vi "Teste_freescale.vi"() -> ()   [LabVIEW 2019]
uses:
  <vilib>/Instr/_visa.llb/VISA Configure Serial Port (Instr).vi
panel:
  in  "Escrever para a \nplaca em\n decimal":string
  out "hexadecimal para a placa":string
  out "leitura da placa":string
  in  "VISA resource name":refnum<visa-resource-name>
  in  "stop":bool
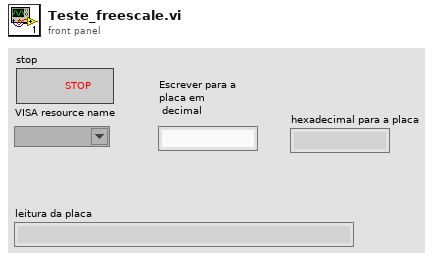
[diagram p1: front panel]
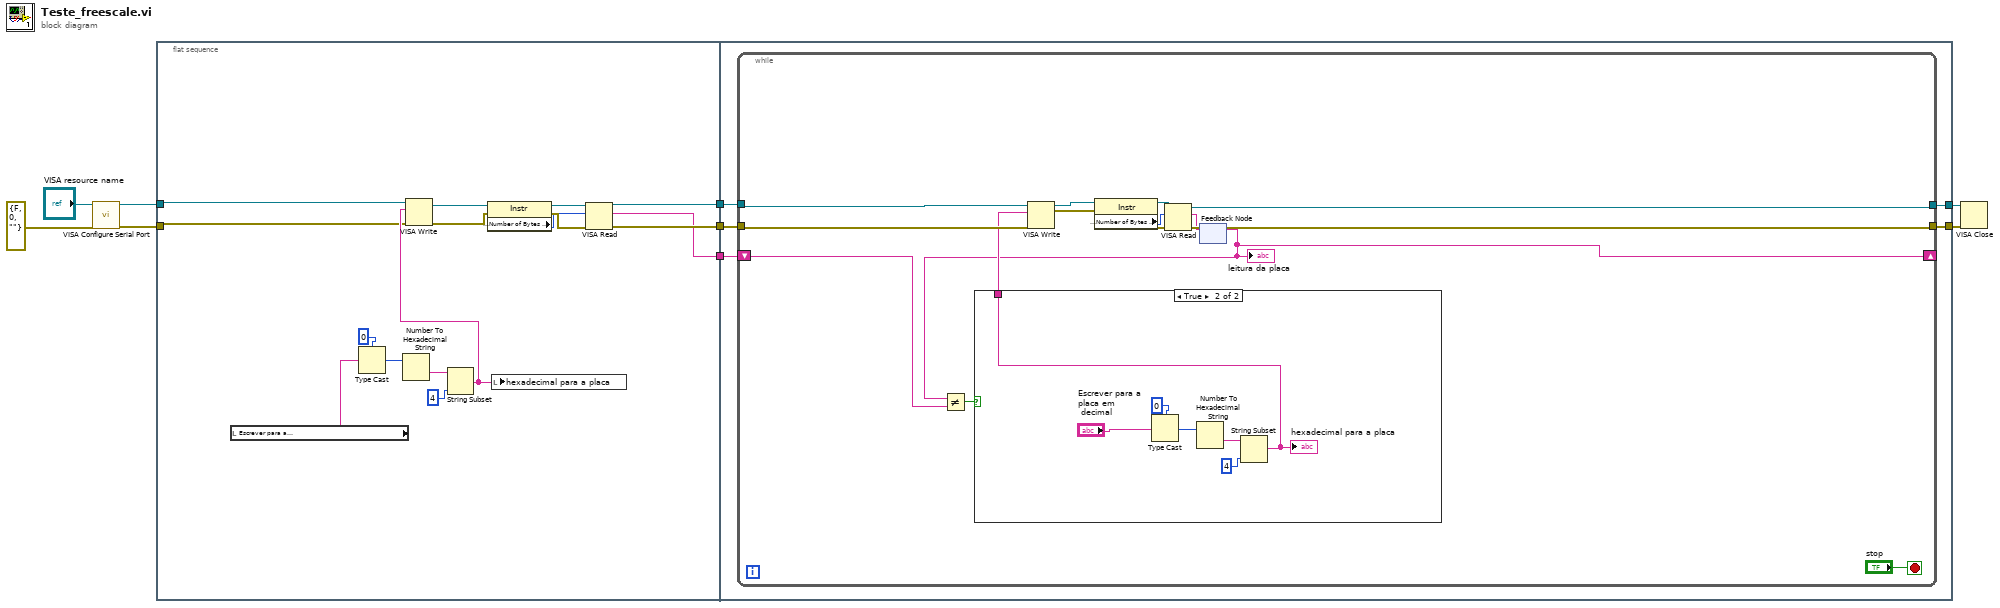
[diagram p0: block diagram]
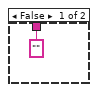
[diagram p2: hidden frame]
diagram:
  n1 = call-poly "VISA Configure Serial Port"("VISA resource name"="VISA resource name", "error in (no error)"=errorcluster {"status"=FALSE, "code"=0, "source"=""}) -> ("VISA resource name out"=w8:refnum<visa-resource-name>, "error out"=w7:errorcluster)  [unwired: 12 in]
  n2 = flat-sequence {
    tunnel: w7 -> [w19]
    tunnel: w8 -> [w18]
    tunnel: [w11] -> w3
    tunnel: [w12] -> w2
    tunnel: [w10] -> w1
    tunnel: [w28] -> w5
    tunnel: [w27] -> w4
    tunnel: w3 -> [w29]
    tunnel: w2 -> [w30]
    tunnel: w1 -> [w26]
    frame #0 {
      n3 = local read "Escrever para a \nplaca em\n decimal"() -> (w21:string)
      n4 = Type Cast(type=0, x=w21) -> (*(type *) &x=w23:i32)
      n5 = Number To Hexadecimal String(2:w23) -> (0:w24:string)  [unwired: 1 in]
      n6 = String Subset(string=w24, length (rest)=4 ("length (rest)")) -> (substring=w20:string)  [unwired: 1 in]
      n7 = VISA Write(VISA resource name=w18, write buffer=w20, error in (no error)=w19) -> (VISA resource name out=w16:refnum<visa-resource-name>, error out=w15:errorcluster)  [unwired: 1 out]
      n8 = property class="Instr"(reference=w16, error in=w15) -> (reference out=w17:refnum<visa-resource-name>, error out=w14:errorcluster, "Serial Settings:Number of Bytes at Serial Port"=w13:u32)
      n9 = local write "hexadecimal para a placa"(w20) -> ()
      n10 = VISA Read(VISA resource name=w17, byte count=w13, error in (no error)=w14) -> (VISA resource name out=w12:refnum<visa-resource-name>, read buffer=w10:string, error out=w11:errorcluster)  [unwired: 1 out]
    }
    frame #1 {
      n11 = while {
        tunnel: w30 -> [w44]
        tunnel: w29 -> [w43]
        tunnel: [w42] -> w28
        tunnel: [w41] -> w27
        shift-right: [w31] -> _
        shift-left: w26 -> [w33]
        stop <- "stop" stop-if-true
        n12 = feedback #1() -> (w31:string)  [unwired: 1 in]
        "leitura da placa" <- w31
        n13 = Not Equal?(x=w31, y=w33) -> (x != y?=w34:bool)
        n14 = case shown="True" w34 {
          tunnel: ["" w47] -> w35
          frame False {
          }
          frame True {
            n15 = Type Cast(type=0, x="Escrever para a \nplaca em\n decimal") -> (*(type *) &x=w50:i32)
            n16 = Number To Hexadecimal String(2:w50) -> (0:w49:string)  [unwired: 1 in]
            n17 = String Subset(string=w49, length (rest)=4 ("length (rest)")) -> (substring=w47:string)  [unwired: 1 in]
            "hexadecimal para a placa" <- w47
          }
        }
        n18 = VISA Write(VISA resource name=w44, write buffer=w35, error in (no error)=w43) -> (VISA resource name out=w40:refnum<visa-resource-name>, error out=w38:errorcluster)  [unwired: 1 out]
        n19 = property class="Instr"(reference=w40, error in=w38) -> (reference out=w37:refnum<visa-resource-name>, error out=w39:errorcluster, "Serial Settings:Number of Bytes at Serial Port"=w36:u32)
        n20 = VISA Read(VISA resource name=w37, byte count=w36, error in (no error)=w39) -> (VISA resource name out=w42:refnum<visa-resource-name>, read buffer=w32:string, error out=w41:errorcluster)  [unwired: 1 out]
        n21 = feedback-in #1(w32) -> ()
      }
    }
  }
  n22 = VISA Close(VISA resource name=w5, error in (no error)=w4) -> ()  [unwired: 1 out]
